vi "VSG_SET_RF_REF_1.00.vi"(6 "POWER REF ON/OFF":bool=TRUE, 8 "error in":errorcluster {"code" format="%.0x"}, 9 "Level":dbl, 10 "Level (str)":string, 11 "Session In":refnum<visa-resource-name>="GPIB0::18::INSTR") -> (0 "error out":errorcluster {"code" format="%.0x"}, 3 "Session Out":refnum<visa-resource-name>)   [LabVIEW 2018]
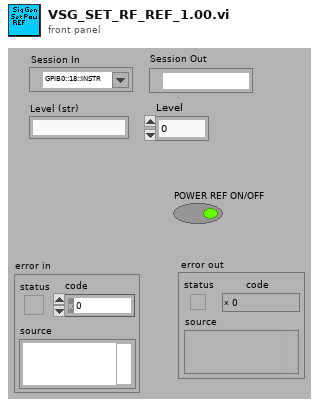
[diagram p1: front panel]
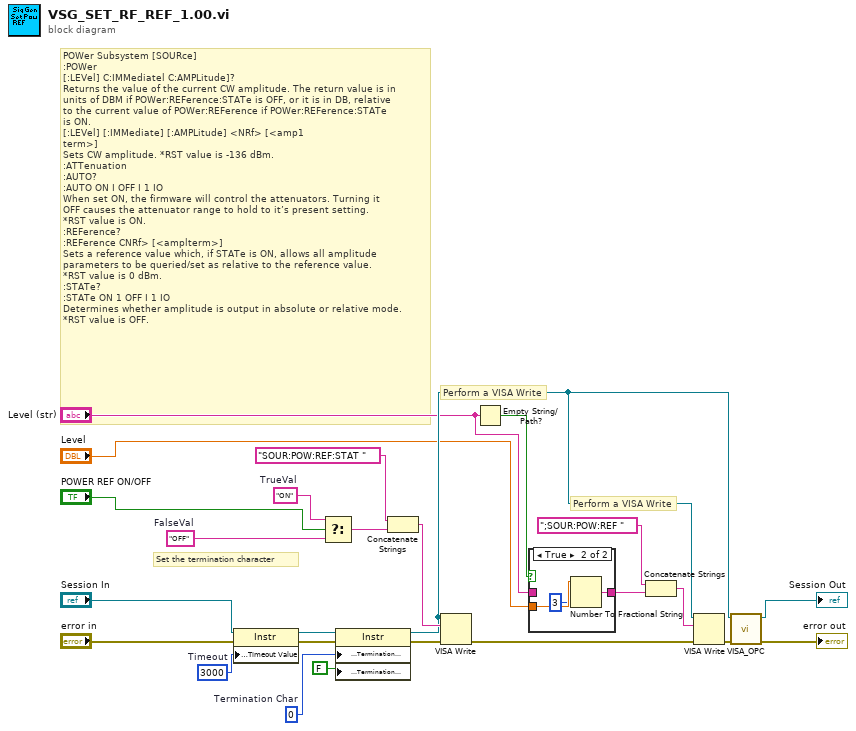
[diagram p0: block diagram]
diagram:
  w18 = u8 0  # Termination Char
  w22 = u32 3000  # Timeout
  w23 = "OFF"  # FalseVal
  w24 = "ON"  # TrueVal
  # "Perform a VISA Write"
  # "Perform a VISA Write"
  # "Set the termination character"
  # "POWer Subsystem [SOURce]\n:POWer\n[:LEVel] C:IMMediatel C:AMPLitude]?\nReturns the value of the current CW amplitude. The return value is in\nunits of DBM if POWer:REFerence:STATe is OFF, or it is in DB, relative\nto the current value of POWer:REFerence if POWer:REFerence:STATe\nis ON.\n[:LEVel] [:IMMediate] [:AMPLitude] <NRf> [<amp1\nterm>]\nSets CW amplitude. *RST value is -136 dBm.\n:ATTenuation\n:AUTO?\n:AUTO ON I OFF I 1 IO\nWhen set ON, the firmware will control the attenuators. Turning it\nOFF causes the attenuator range to hold to it’s present setting.\n*RST value is ON.\n:REFerence?\n:REFerence CNRf> [<amplterm>]\nSets a reference value which, if STATe is ON, allows all amplitude\nparameters to be queried/set as relative to the reference value.\n*RST value is 0 dBm.\n:STATe?\n:STATe ON 1 OFF I 1 IO\nDetermines whether amplitude is output in absolute or relative mode.\n*RST value is OFF."
  n1 = property class="Instr"(reference="Session In", error in="error in", "General Settings:Timeout Value"=w22) -> (reference out=w17:refnum<visa-resource-name>, error out=w20:errorcluster)
  n2 = Select(t=w24, s="POWER REF ON/OFF", f=w23) -> (s? t:f=w15:string)
  n3 = property class="Instr"(reference=w17, error in=w20, "Message Based Settings:Termination Character"=w18, "Message Based Settings:Termination Character Enable"=FALSE ("enable")) -> (reference out=w9:refnum<visa-resource-name>, error out=w19:errorcluster)
  n4 = Concatenate Strings("SOUR:POW:REF:STAT " ("staticText"), w15) -> (w12:string)
  n5 = VISA Write(VISA resource name=w9, write buffer=w12, error in (no error)=w19) -> (error out=w13:errorcluster)  [unwired: 2 out]
  n6 = Empty String/Path?(string/path="Level (str)") -> (empty?=w1:bool)
  n7 = case shown="True" w1 {
    tunnel: "Level" -> [_ w29]
    tunnel: [w26 w28] -> w3
    tunnel: "Level (str)" -> [w26 _]
    frame False {
    }
    frame True {
      n8 = Number To Fractional String(number=w29, precision (6)=i16 3) -> (F-format string=w28:string)  [unwired: 2 in]
    }
  }
  n9 = Concatenate Strings(";SOUR:POW:REF " ("staticText"), w3) -> (w10:string)
  n10 = VISA Write(VISA resource name=w9, write buffer=w10, error in (no error)=w13) -> (error out=w6:errorcluster)  [unwired: 2 out]
  n11 = call "VISA_OPC.vi"("error in"=w6, "Session In"=w9) -> ("error out"=→"error out":errorcluster, "Session Out"=→"Session Out":refnum<visa-resource-name>)  [unwired: 7 in, 1 out]
